vi "Broadcast Single Message.vi"(8 "error in (no error)":errorcluster, 9 "Mail Strategy In":refnum<class "Mail Strategy.lvclass">, 10 "Message In":refnum<class "Message.lvclass">, 11 "Messenger in":refnum<class "Simple Tree Queue Messenger.lvclass">) -> (0 "error out":errorcluster, 3 "Messenger out":refnum<class "Simple Tree Queue Messenger.lvclass">)   [LabVIEW 2024, in "Simple Tree Queue Messenger.lvclass"]
uses:
  Simple Tree Queue Messenger.lvclass
  Ancestor Class/Message/Message.lvclass
  Ancestor Class/Messenger/Mail Strategy/Mail Strategy.lvclass
  Simple Tree Queue Messenger.lvclass/Simple Tree Queue Messenger.ctl
  Ancestor Class/Messenger/Messenger Composite/Messenger Composite.lvclass/Messenger Composite.ctl
  Ancestor Class/Messenger/Messenger Composite/Public Data/Read Nodes.vi
  Ancestor Class/Messenger/Messenger/Messenger.lvclass
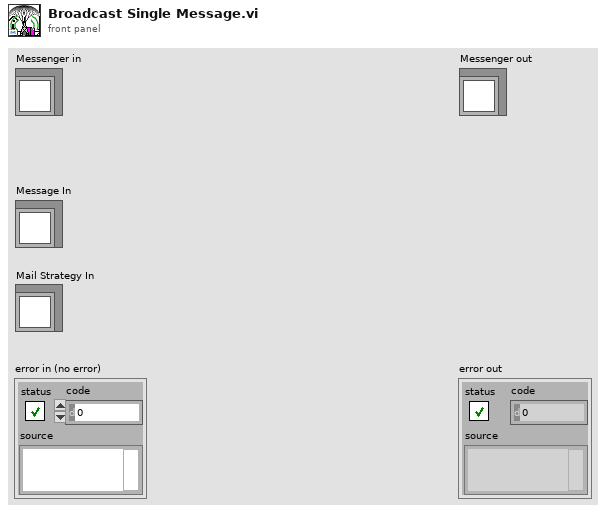
[diagram p1: front panel]
types:
  T1 = typedef "Message Queue.ctl" = refnum<queue>
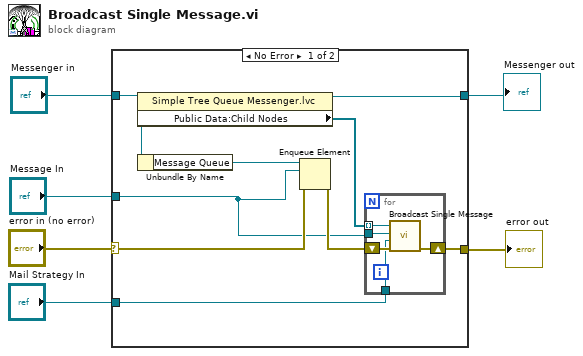
[diagram p0: block diagram]
diagram:
  n1 = case shown="No Error" "error in (no error)" {
    selector: "error in (no error)" -> [w14 w22]
    tunnel: [w12 w22] -> w2
    tunnel: [w9 w21] -> w3
    tunnel: "Messenger in" -> [w10 w21]
    tunnel: "Message In" -> [w11 _]
    tunnel: "Mail Strategy In" -> [w7 _]
    frame No Error {
      n2 = property class="Simple Tree Queue Messenger.lvc"(reference=w10) -> (reference out=w9:refnum<class "Simple Tree Queue Messenger.lvclass">, "Public Data:Child Nodes"=w8:refnum<class "Messenger.lvclass">[])  [unwired: 1 in, 1 out]
      n3 = Unbundle By Name(w10) -> ("Message Queue"=w15:T1)
      n4 = Enqueue Element(queue=w15, element=w11, error in (no error)=w14) -> (error out=w13:errorcluster)  [unwired: 1 in, 2 out]
      n5 = for {
        shift-right: [w17] -> w12
        shift-left: w13 -> [w18]
        tunnel: w8 -> [w20] mode=indexing
        tunnel: w11 -> [w19]
        tunnel: w7 -> [w16]
        n6 = call-dynamic "Broadcast Single Message.vi"("error in (no error)"=w18, "Mail Strategy In"=w16, "Message In"=w19, "Messenger in"=w20) -> ("error out"=w17:errorcluster)  [unwired: 6 in, 1 out]
      }
    }
    frame Error {
    }
  }
  "error out" <- w2
  "Messenger out" <- w3
